vi "IHM_GetControlsRefs.vi"(8 "Error In":errorcluster caption="Entrée d'erreur", 11 "chemin du VI":path) -> (0 "Error Out":errorcluster caption="Sortie d'erreur", 3 "CtrlsRefs_OUT":T1[](array[typedef]))   [LabVIEW 2013]
uses:
  CTL/CtrlRef.ctl
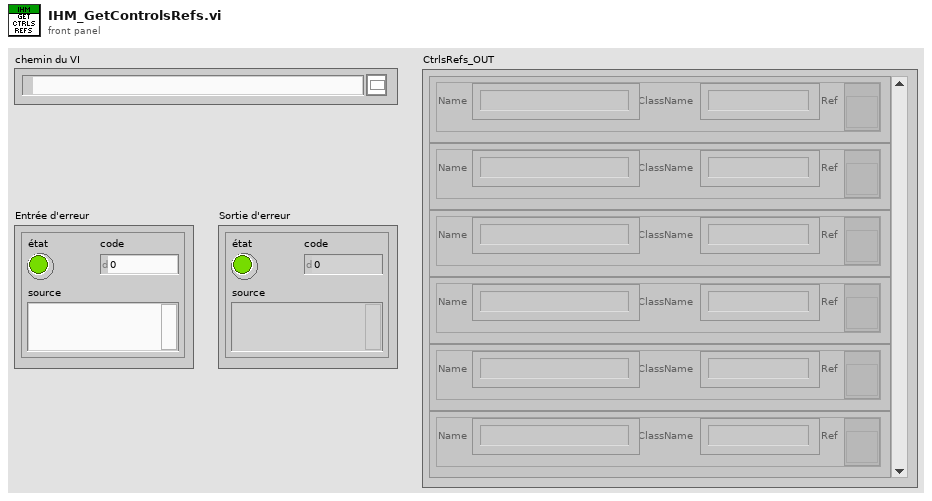
[diagram p1: front panel]
types:
  T1 = typedef "CtrlRef.ctl" = cluster{"Name":string, "Ref":refnum<vi>, "ClassName":string}
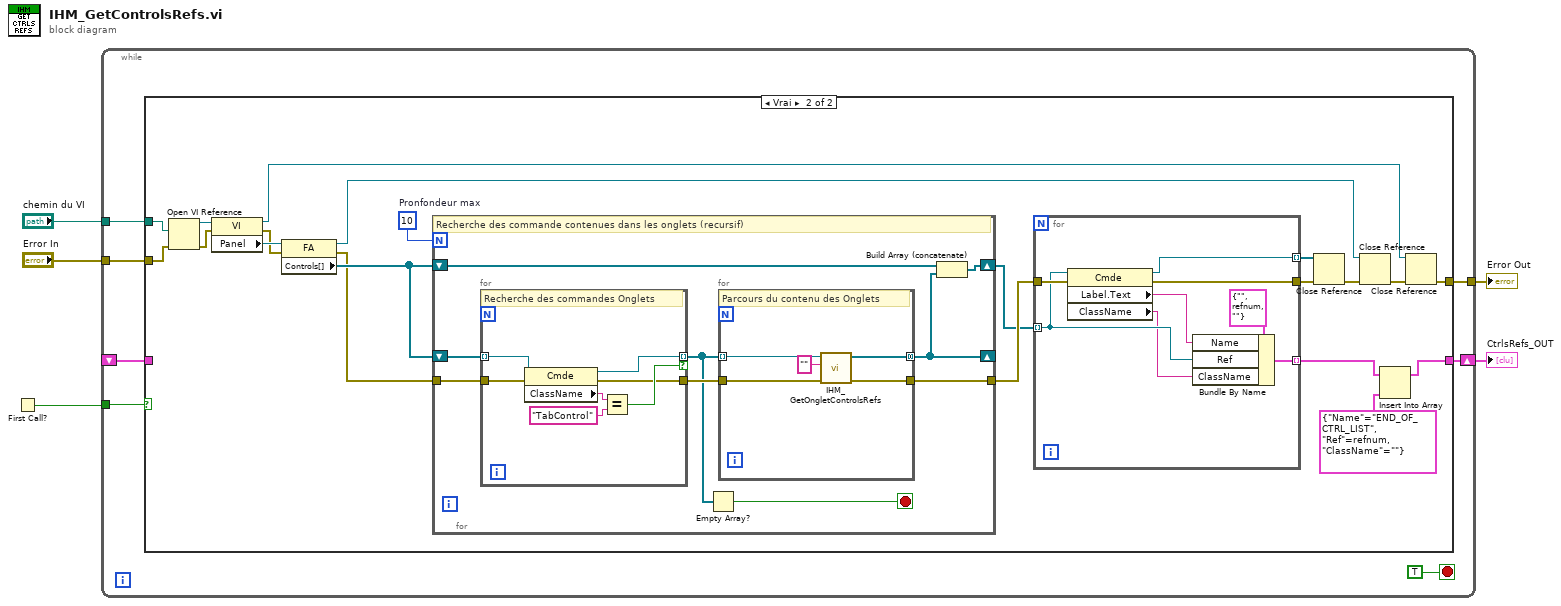
[diagram p0: block diagram]
diagram:
  n1 = First Call?() -> (First Call?: T/F=w5:bool)
  n2 = while {
    tunnel: [w12] -> w3
    tunnel: "Error In" -> [w11]
    tunnel: w5 -> [w10]
    shift-right: [w8] -> w1
    shift-left: _ -> [w7]
    tunnel: "chemin du VI" -> [w6]
    stop <- TRUE stop-if-true
    n3 = case shown="Vrai" w10 {
      tunnel: w11 -> [w13 w24]
      tunnel: [w13 w28] -> w12
      tunnel: [w14 w15] -> w8
      tunnel: w7 -> [w14 _]
      tunnel: w6 -> [_ w26]
      frame False {
      }
      frame True {
        w22 = 10  # Pronfondeur max
        n4 = Open VI Reference(vi path=w26, error in (no error)=w24) -> (vi reference=w27:refnum<vi>, error out=w25:errorcluster)  [unwired: 4 in]
        n5 = property class="VI"(reference=w27, error in=w25) -> (reference out=w30:refnum<vi>, error out=w34:errorcluster, "Panel"=w35:refnum<vi>)
        n6 = property class="FA"(reference=w35, error in=w34) -> (reference out=w31:refnum<vi>, error out=w20:errorcluster, "Controls[]"=w21:refnum<vi>[])
        n7 = for {
          N: w22 -> [_]
          tunnel: w20 -> [w44]
          shift-right: [w37] -> _
          shift-left: w21 -> [w39]
          tunnel: [w36] -> w19
          shift-right: [w38] -> w18
          shift-left: w21 -> [w40]
          stop <- w41 stop-if-true
          # "Recherche des commande contenues dans les onglets (recursif)"
          n8 = for {
            tunnel: w39 -> [w56] mode=indexing
            tunnel: w44 -> [w55]
            tunnel: [w50] -> w43
            tunnel: [w51] -> w42 mode=indexing if=w52
            # "Recherche des commandes Onglets"
            n9 = property class="Cmde"(reference=w56, error in=w55) -> (reference out=w51:refnum<vi>, error out=w50:errorcluster, "ClassName"=w54:string)
            n10 = Equal?(x=w54, y="TabControl") -> (x = y?=w52:bool)
          }
          n11 = Empty Array?(array=w42) -> (empty?=w41:bool)
          n12 = for {
            tunnel: w43 -> [w48]
            tunnel: w42 -> [w49] mode=indexing
            tunnel: [w46] -> w37 mode=concatenating
            tunnel: [w45] -> w36
            # "Parcours du contenu des Onglets"
            n13 = call "IHM_GetOngletControlsRefs.vi"("Error In"=w48, "PageName"="", "OngletRef"=w49) -> ("Error Out"=w45:errorcluster, "ControlsOnPage"=w46:refnum<vi>[])  [unwired: 6 in, 1 out]
          }
          n14 = Build Array (concatenate)(w40, w37) -> (w38:refnum<vi>[])
        }
        n15 = for {
          tunnel: w18 -> [w59] mode=indexing
          tunnel: [w60] -> w17 mode=indexing
          tunnel: w19 -> [w64]
          tunnel: [w63] -> w33
          tunnel: [w62] -> w32 mode=indexing
          n16 = property class="Cmde"(reference=w59, error in=w64) -> (reference out=w62:refnum<vi>, error out=w63:errorcluster, "Label.Text"=w57:string, "ClassName"=w58:string)
          n17 = Bundle By Name(cluster=T1 {"Name"="", "Ref"=refnum, "ClassName"=""} ("CtrlRef"), "Name"=w57, "Ref"=w59, "ClassName"=w58) -> (w60:T1)
        }
        n18 = Close Reference(reference=w32, error in (no error)=w33) -> (error out=w23:errorcluster)
        n19 = Close Reference(reference=w31, error in (no error)=w23) -> (error out=w29:errorcluster)
        n20 = Insert Into Array(array=w17, new element=T1 {"Name"="END_OF_CTRL_LIST", "Ref"=refnum, "ClassName"=""} ("CtrlRef")) -> (w15:T1[])  [unwired: 1 in]
        n21 = Close Reference(reference=w30, error in (no error)=w29) -> (error out=w28:errorcluster)
      }
    }
  }
  "Error Out" <- w3
  "CtrlsRefs_OUT" <- w1
